vi "Calc Saturated Ampl.vi"(11 "Waveform":dbl[](array[numeric])) -> (0 "RMS Amplitude":dbl, 1 "Rising":i32, 2 "1/2 Period":i32, 3 "Falling":i32, 4 "Sat. Ind":u64, 5 "Peak Amplitude":dbl)   [LabVIEW 2017]
uses:
  <vilib>/measure/mamon.llb/Trigger Detection for 1 Channel.vi
  <vilib>/measure/NI_MAPro.lvlib
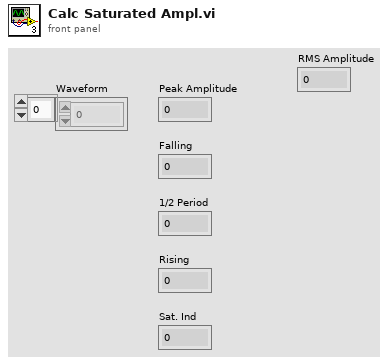
[diagram p1: front panel]
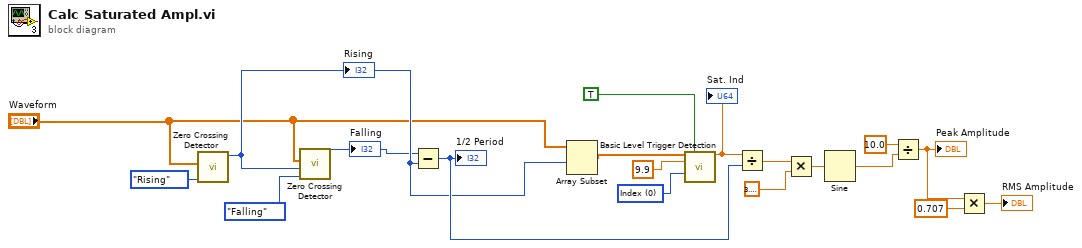
[diagram p0: block diagram]
diagram:
  w9 = u16 0 items=["Index", "Time"] ("location mode")
  n1 = call "Zero Crossing Detector.vi"("Direction"=enum16{"Rising", "Falling"}."Rising", "Y"="Waveform") -> ("X"=w12:i32)  [unwired: 9 in]
  "Rising" <- w12
  n2 = call "Zero Crossing Detector.vi"("Direction"=enum16{"Rising", "Falling"}."Falling", "offset"=w12, "Y"="Waveform") -> ("X"=w6:i32)  [unwired: 8 in]
  "Falling" <- w6
  n3 = Subtract(x=w6, y=w12) -> (x-y=w14:i32)
  "1/2 Period" <- w14
  n4 = Array Subset(array="Waveform", index=w12) -> (w11:dbl[])  [unwired: 1 in]
  n5 = call-poly <vilib>:"Basic Level Trigger Detection.vi"("signal in"=w11, "reset"=TRUE, "level"=9.9, "location mode"=w9) -> ("trigger location"=w13:dbl)  [unwired: 9 in, 2 out]
  "Sat. Ind" <- w13
  n6 = Divide(x=w13, y=w14) -> (x/y=w15:dbl)
  n7 = Multiply(x=w15, y=3.141592653589793) -> (x*y=w17:dbl)
  n8 = Sine(x=w17) -> (sin(x)=w19:dbl)
  n9 = Divide(x=10.0, y=w19) -> (x/y=w3:dbl)
  "Peak Amplitude" <- w3
  n10 = Multiply(x=w3, y=0.707) -> (x*y=→"RMS Amplitude":dbl)
